vi "logl.vi"(9 "para2":cluster{}, 10 "format":string, 11 "level":u32(ring) items=["APDM_LL_ALL", "APDM_LL_DEBUG", "APDM_LL_INFO", "APDM_LL_WARNING", "APDM_LL_ERROR", "APDM_LL_NONE"]) -> (3 "function return":i32)   [LabVIEW 2019, in "apdm.lvlib"]
doc: "APDM_EXPORT int apdm_logl(const enum APDM_Logging_Level level, const char *format, ...);"
uses:
  apdm.lvlib
  Lee Lab/CP FES Walking 2018/Code/Working/LabVIEW/apdm.dll
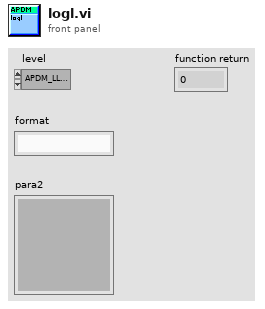
[diagram p1: front panel]
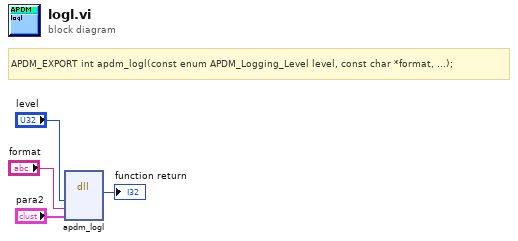
[diagram p0: block diagram]
diagram:
  # "APDM_EXPORT int apdm_logl(const enum APDM_Logging_Level level, const char *format, ...);"
  n1 = dll-call lib="C:/Users/jfalesi/Dropbox/Lee Lab/CP FES Walking 2018/Code/Working/LabVIEW/apdm.*" fn="apdm_logl"("level"="level", "format"="format", "para2"="para2") -> (→"function return":i32)  [unwired: 6 in, 2 out]
